vi "Set Scalar Configuration.vi"(8 "error in (no error)":errorcluster, 9 "index":i32, 10 "group configuration":T1={"name"="Group", "direction"=enum."Tx", "cycle timing"={"priority"=100, "decimation"=1, "offset"=0}, "timeout behavior"=enum."Increment Late Count", "convert buffers"=FALSE}, 11 "Core Groups Configuration in":refnum<class "Core Groups Configuration.lvclass">) -> (0 "error out":errorcluster, 3 "Core Groups Configuration out":refnum<class "Core Groups Configuration.lvclass">)   [LabVIEW 2017, in "DSF Core.lvlib" / "Core Groups Configuration.lvclass"]
uses:
  Core Groups Configuration.lvclass
  Configuration.ctl
  Typedefs/DSF Direction.ctl
  Typedefs/DSF Timing Info.ctl
  Typedefs/DSF Timeout Behavior.ctl
  Core Groups Configuration.lvclass/Core Groups Configuration.ctl
  DSF Core.lvlib
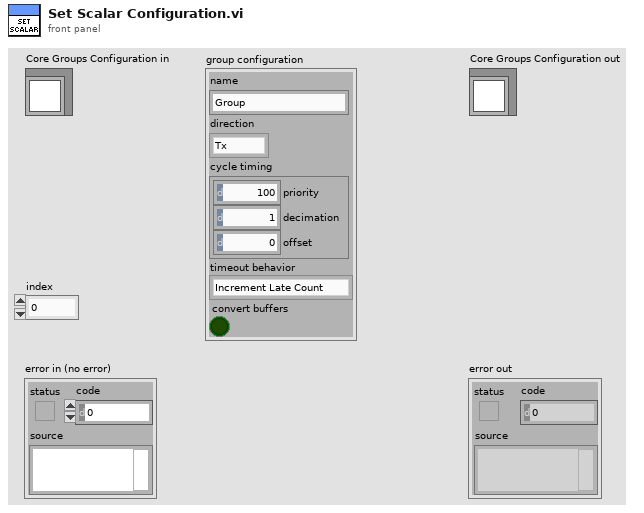
[diagram p1: front panel]
types:
  T1 = typedef "DSF Core.lvlib/Core Groups Configuration.lvclass/Configuration.ctl" = cluster{"name":string, "direction":T2, "cycle timing":T3, "timeout behavior":T4, "convert buffers":bool}
  T2 = typedef "DSF Core.lvlib/DSF Direction.ctl" = enum8{"Tx", "Rx"}
  T3 = typedef "DSF Core.lvlib/DSF Timing Info.ctl" = cluster{"priority":u64, "decimation":u64, "offset":u64}
  T4 = typedef "DSF Core.lvlib/DSF Timeout Behavior.ctl" = enum8{"Increment Late Count", "Throw Error"}
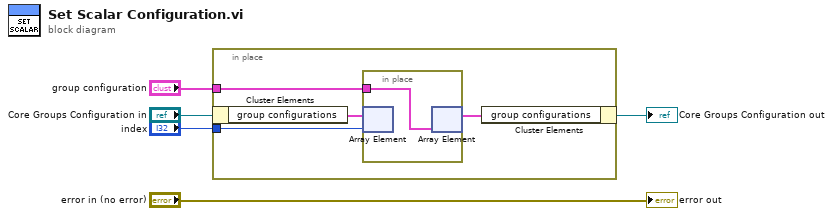
[diagram p0: block diagram]
diagram:
  n1 = in-place {
    in-place-border: "index" -> [w8]
    in-place-border: "group configuration" -> [w7]
    n2 = in-place-cluster #1("Core Groups Configuration in") -> ("group configurations"=w9:T1[])
    n3 = in-place {
      in-place-border: w7 -> [w10]
      n4 = in-place-array #2(w9, w8) -> ()  [unwired: 1 out]
      n5 = in-place-array #2(w10) -> (w6:T1[])  [unwired: 1 out]
    }
    n6 = in-place-cluster #1("group configurations"=w6) -> (→"Core Groups Configuration out":refnum<class "Core Groups Configuration.lvclass">)
  }
  "error out" <- "error in (no error)"
